vi "Start Discovery.vi"(8 "error in (no error)":errorcluster, 11 "Vecto in":refnum<class "Vecto.lvclass">) -> (0 "error out":errorcluster, 3 "Vecto out":refnum<class "Vecto.lvclass">)   [LabVIEW 2020, in "Vecto.lvlib" / "Vecto.lvclass"]
uses:
  Vecto.lvclass
  DiscoveryService/DiscoveryService.lvclass
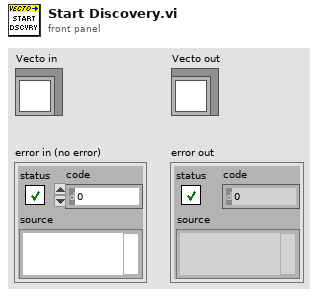
[diagram p1: front panel]
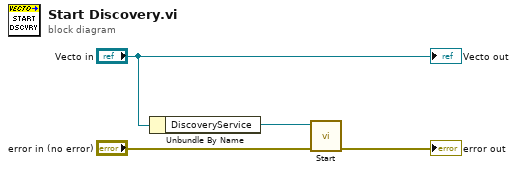
[diagram p0: block diagram]
diagram:
  n1 = Unbundle By Name("Vecto in") -> ("DiscoveryService"=w4:refnum<class "DiscoveryService.lvclass">)
  n2 = call "Start.vi"("error in (no error)"="error in (no error)", "DiscoveryService in"=w4) -> ("error out"=→"error out":errorcluster)  [unwired: 8 in, 1 out]
  "Vecto out" <- "Vecto in"
